vi "square plot.vi"() -> ()   [LabVIEW 2020]
panel:
  out "Waveform Graph 2":i32[](graph)
  out "Waveform Graph":i32[](graph)
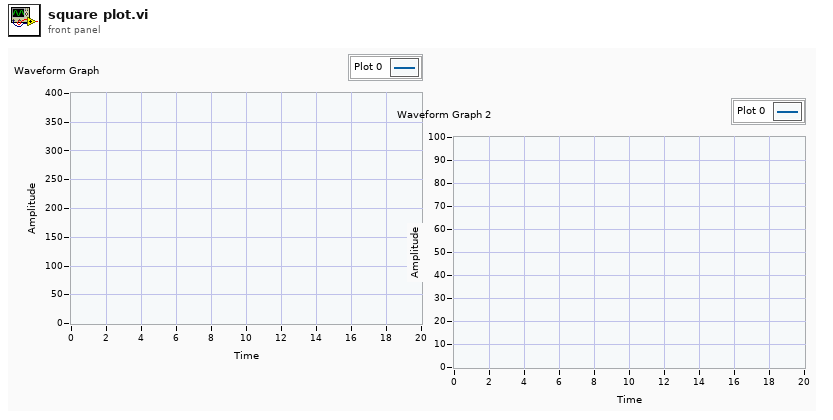
[diagram p1: front panel]
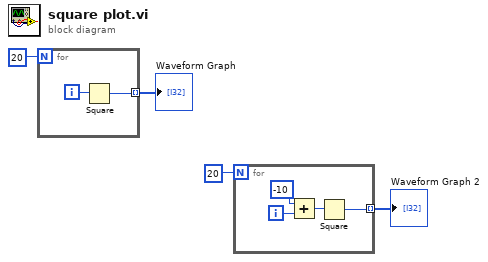
[diagram p0: block diagram]
diagram:
  n1 = for {
    N: 20 -> [_]
    tunnel: [w5] -> w4 mode=indexing
    i -> [w6]
    n2 = Square(x=w6) -> (x^2=w5:i32)
  }
  "Waveform Graph" <- w4
  n3 = for {
    N: 20 -> [_]
    tunnel: [w10] -> w2 mode=indexing
    i -> [w8]
    n4 = Add(x=-10, y=w8) -> (x+y=w9:i32)
    n5 = Square(x=w9) -> (x^2=w10:i32)
  }
  "Waveform Graph 2" <- w2
